vi "根据直线计算旋转矩形.vi"(10 "Img in":T2, 11 "Straight Edge (Y1)":T3) -> (3 "ROI Descriptor":T1 {"Contours"."Type" items=["No Selection", "Point", "Line", "Rectangle", "Oval", "Polygon", "Freehand Region", "Annulus", "Unused2", "Unused3", "Broken Line", "Freehand Line", "Rotated Rectangle"]})   [LabVIEW 2014]
uses:
  <vilib>/vision/Image Controls.llb/IMAQ Image.ctl
  <vilib>/Analysis/coordinate.llb/2D Cartesian Coordinate Rotation (Scalar).vi
  <vilib>/Analysis/NI_AALPro.lvlib
panel:
  out "左上角点":cluster{"X":sgl, "Y":sgl}
  out "左下角点":cluster{"X":sgl, "Y":sgl}
  out "右上角点":cluster{"X":sgl, "Y":sgl}
  out "右下角点":cluster{"X":sgl, "Y":sgl}
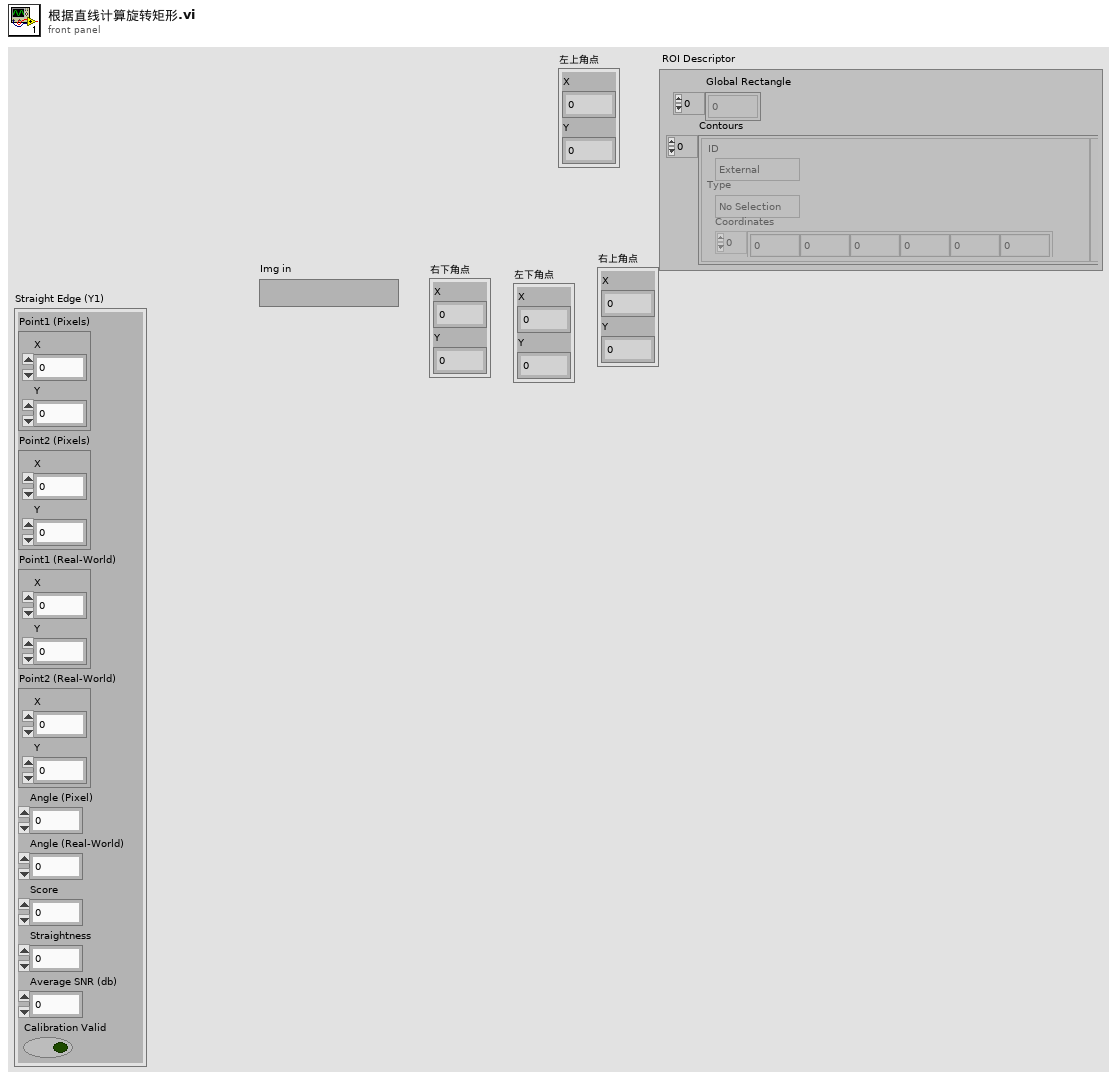
[diagram p1: front panel]
types:
  T1 = typedef "ROI Descriptor" = cluster{"Global Rectangle":i32[], "Contours":cluster{"ID":enum32{"External", "Internal"}, "Type":u32, "Coordinates":i32[]}[]}
  T2 = typedef "IMAQ Image.ctl" = refnum<image>
  T3 = cluster{"Point1 (Pixels)":cluster{"X":sgl, "Y":sgl}, "Point2 (Pixels)":cluster{"X":sgl, "Y":sgl}, "Point1 (Real-World)":cluster{"X":sgl, "Y":sgl}, "Point2 (Real-World)":cluster{"X":sgl, "Y":sgl}, "Angle (Pixel)":dbl, "Angle (Real-World)":dbl, "Score":dbl, "Straightness":dbl, "Average SNR (db)":dbl, "Calibration Valid":bool}
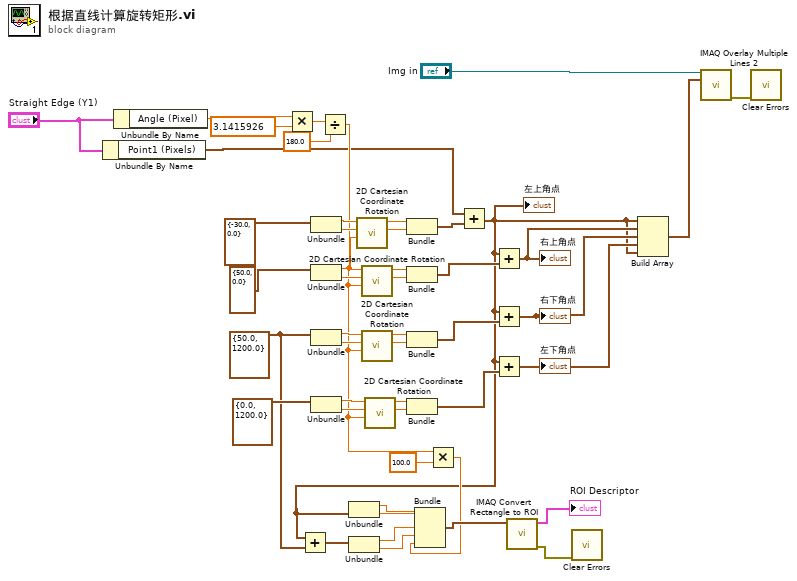
[diagram p0: block diagram]
diagram:
  w14 = cluster{"X":sgl, "Y":sgl} {"X"=50.0, "Y"=1200.0} ("y")
  n1 = Unbundle By Name("Straight Edge (Y1)") -> ("Point1 (Pixels)"=w2:cluster{"X":sgl, "Y":sgl})
  n2 = Unbundle By Name("Straight Edge (Y1)") -> ("Angle (Pixel)"=w25:dbl)
  n3 = Multiply(x=w25, y=3.1415926) -> (x*y=w24:dbl)
  n4 = Unbundle(cluster{"X":sgl, "Y":sgl} {"X"=-30.0, "Y"=0.0} ("y")) -> ("X"=w18:sgl, "Y"=w19:sgl)
  n5 = Unbundle(cluster{"X":sgl, "Y":sgl} {"X"=50.0, "Y"=0.0} ("y")) -> ("X"=w46:sgl, "Y"=w45:sgl)
  n6 = Unbundle(w14) -> ("X"=w39:sgl, "Y"=w40:sgl)
  n7 = Unbundle(cluster{"X":sgl, "Y":sgl} {"X"=0.0, "Y"=1200.0} ("y")) -> ("X"=w37:sgl, "Y"=w36:sgl)
  n8 = Divide(x=w24, y=180.0) -> (x/y=w5:dbl)
  n9 = call-poly <vilib>:"2D Cartesian Coordinate Rotation.vi"("theta"=w5, "y"=w19, "x"=w18) -> ("y out"=w21:dbl, "x out"=w20:dbl)  [unwired: 6 in, 1 out]
  n10 = call-poly <vilib>:"2D Cartesian Coordinate Rotation.vi"("theta"=w5, "y"=w45, "x"=w46) -> ("y out"=w43:dbl, "x out"=w44:dbl)  [unwired: 6 in, 1 out]
  n11 = call-poly <vilib>:"2D Cartesian Coordinate Rotation.vi"("theta"=w5, "y"=w40, "x"=w39) -> ("y out"=w42:dbl, "x out"=w41:dbl)  [unwired: 6 in, 1 out]
  n12 = call-poly <vilib>:"2D Cartesian Coordinate Rotation.vi"("theta"=w5, "y"=w36, "x"=w37) -> ("y out"=w34:dbl, "x out"=w35:dbl)  [unwired: 6 in, 1 out]
  n13 = Bundle("x out"=w20, "y out"=w21) -> (w17:cluster{"x out":dbl, "y out":dbl})  [unwired: 1 in]
  n14 = Bundle("x out"=w44, "y out"=w43) -> (w33:cluster{"x out":dbl, "y out":dbl})  [unwired: 1 in]
  n15 = Bundle("x out"=w41, "y out"=w42) -> (w32:cluster{"x out":dbl, "y out":dbl})  [unwired: 1 in]
  n16 = Bundle("x out"=w35, "y out"=w34) -> (w31:cluster{"x out":dbl, "y out":dbl})  [unwired: 1 in]
  n17 = Multiply(x=w5, y=100.0) -> (x*y=w3:dbl)
  n18 = Add(x=w2, y=w17) -> (x+y=w1:cluster{dbl, dbl})
  "左上角点" <- w1
  n19 = Add(x=w1, y=w14) -> (x+y=w13:cluster{dbl, dbl})
  n20 = Unbundle(w1) -> (w12:dbl, w11:dbl)
  n21 = Unbundle(w13) -> (w10:dbl, w9:dbl)
  n22 = Bundle(w12, w11, w10, w9, w3) -> (w8:cluster{dbl, dbl, dbl, dbl, dbl})  [unwired: 1 in]
  n23 = Add(x=w1, y=w33) -> (x+y=w29:cluster{dbl, dbl})
  "右上角点" <- w29
  n24 = Add(x=w1, y=w32) -> (x+y=w28:cluster{dbl, dbl})
  "右下角点" <- w28
  n25 = Add(x=w1, y=w31) -> (x+y=w27:cluster{dbl, dbl})
  "左下角点" <- w27
  n26 = call "IMAQ Convert Rectangle to ROI"("Rectangle"=w8) -> ("error out"=w7:errorcluster, "ROI Descriptor"=→"ROI Descriptor":T1)  [unwired: 8 in]
  n27 = call <vilib>:"Clear Errors.vi"("error in (no error)"=w7) -> ()  [unwired: 5 in, 2 out]
  n28 = Build Array(w1, w29, w28, w27, w1) -> (w26:cluster{dbl, dbl}[])
  n29 = call "IMAQ Overlay Multiple Lines 2"("Image"="Img in", "Line End Points"=w26) -> ("error out"=w16:errorcluster)  [unwired: 12 in, 1 out]
  n30 = call <vilib>:"Clear Errors.vi"("error in (no error)"=w16) -> ()  [unwired: 5 in, 2 out]
